vi "Not.vi"(1 "Input":bool) -> (0 "Output":bool)   [LabVIEW 2020, in "Hack.lvlib"]
uses:
  Hack.lvlib
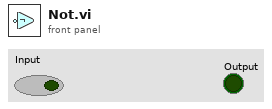
[diagram p1: front panel]
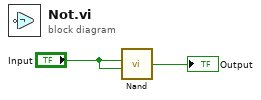
[diagram p0: block diagram]
diagram:
  n1 = call "Nand.vi"("B"="Input", "A"="Input") -> ("Output"=→"Output":bool)  [unwired: 2 in]
